vi "SpawnMediatorActor.vi"(6 "Unified Actor Alias":string, 9 "Core Leaf Actors":refnum<class "Actor.lvclass">[](array[class]), 10 "Actors":refnum<class "Actor.lvclass">[](array[class])) -> (0 "Error out":errorcluster, 2 "Root Unified Actor DVR":refnum<data-value>)   [LabVIEW 2020, in "jettl.lvlib"]
uses:
  jettl.lvlib
  Actor.ctl
  ActorLifetime.ctl
  Message/Message.lvclass
  MessageSet.ctl
  ActorRelation.ctl
  MessageMetadata.ctl
  Message.ctl
  Messages.ctl
  Actor/Actor.lvclass
  BaseActor/BaseActor.lvlib
  ActorType.ctl
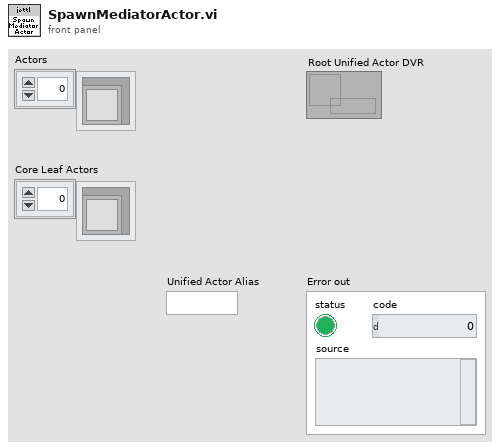
[diagram p1: front panel]
types:
  T1 = typedef "jettl.lvlib/Messages.ctl" = cluster{"Listen":T2, "Tell":T2, "TellSelf":T2, "TellActor":T2}
  T2 = typedef "jettl.lvlib/MessageSet.ctl" = set{refnum<class "Message.lvclass">}
  T3 = typedef "jettl.lvlib/Actor.ctl" = cluster{"Messages":T1, "Alias":string, "Transport":refnum<user-event>, "Address":refnum<event-registration>, "VIRef":refnum<vi>, "ActorType":T4}
  T4 = typedef "jettl.lvlib/ActorType.ctl" = enum16{"Mediator", "Component"}
  T5 = typedef "jettl.lvlib/ActorLifetime.ctl" = enum16{"Init", "Spawn", "Setup", "Teardown Before Running", "Running", "Stop Called", "Stopping With Children", "Stopping Without Children", "Teardown After Running", "Stopped"}
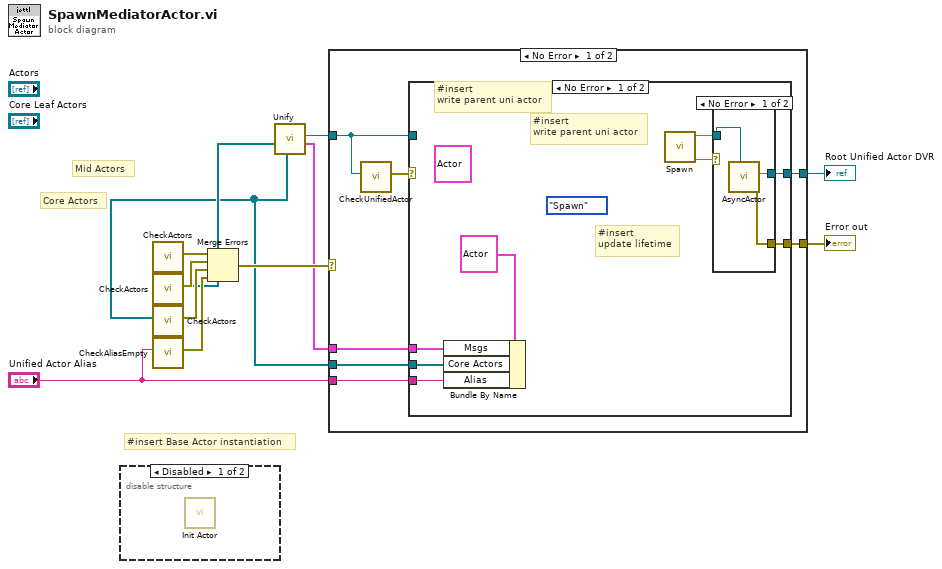
[diagram p0: block diagram]
diagram:
  # "Core Actors"
  # "Mid Actors"
  # "#insert Base Actor instantiation"
  n1 = disable-structure shown="Disabled" {
    frame Disabled {
      n2 = call "Init Actor.vi"() -> ()  [unwired: 11 in, 1 out]
    }
    frame Enabled {
    }
  }
  n3 = call "CheckActors.vi"() -> ("Error"=w7:errorcluster)  [unwired: 11 in]
  n4 = call "CheckActors.vi"() -> ("Error"=w11:errorcluster, "Actors"=w6:refnum<class "Actor.lvclass">[])  [unwired: 10 in]
  n5 = call "CheckActors.vi"() -> ("Error"=w8:errorcluster, "Actors"=w5:refnum<class "Actor.lvclass">[])  [unwired: 10 in]
  n6 = call "CheckAliasEmpty.vi"("Alias"="Unified Actor Alias") -> ("Error"=w10:errorcluster)  [unwired: 10 in]
  n7 = Merge Errors(w7, w11, w8, w10) -> (w12:errorcluster)
  n8 = call "Unify.vi"("Core Actors"=w5, "Mid Actors"=w6) -> ("Msgs"=w3:T1, "Unified Actor"=w2:refnum<class "Actor.lvclass">)  [unwired: 7 in, 1 out]
  n9 = case shown="No Error" w12 {
    selector: w12 -> [_ w37]
    tunnel: [w19 w37] -> w1
    tunnel: [w18 _] -> w4
    tunnel: "Unified Actor Alias" -> [w17 _]
    tunnel: w5 -> [w13 _]
    tunnel: w3 -> [w15 _]
    tunnel: w2 -> [w14 _]
    frame No Error {
      n10 = call "CheckUnifiedActor.vi"("Unified Actor"=w14) -> ("Error"=w16:errorcluster)  [unwired: 10 in]
      n11 = case shown="No Error" w16 {
        selector: w16 -> [_ w36]
        tunnel: [w31 w36] -> w19
        tunnel: [w30 _] -> w18
        tunnel: w17 -> [w29 _]
        tunnel: w15 -> [w27 _]
        tunnel: w14 -> [w22 _]
        tunnel: w13 -> [w23 _]
        frame No Error {
          w21 = ActorLifetime."Spawn" ("Lifetime")
          (unwired) T3 {"Messages"={"Listen"={}, "Tell"={}, "TellSelf"={}, "TellActor"={}}, "Alias"="", "Transport"=refnum, "Address"=refnum, "VIRef"=refnum, "ActorType"=enum."Mediator"} ("Parent Actor Attributes")
          # "#insert\nupdate lifetime"
          # "#insert\nwrite parent uni actor"
          # "#insert\nwrite parent uni actor"
          n12 = Bundle By Name(cluster=T3 {"Messages"={"Listen"={}, "Tell"={}, "TellSelf"={}, "TellActor"={}}, "Alias"="", "Transport"=refnum, "Address"=refnum, "VIRef"=refnum, "ActorType"=enum."Mediator"} ("Attributes"), "Msgs"=w27, "Core Actors"=w23, "Alias"=w29) -> (w26:T3)
          n13 = call-dynamic "Spawn.vi"() -> (0:w24, 3:w25, 11:w20)  [unwired: 7 in, 2 out]
          n14 = case shown="No Error" w24 {
            selector: w24 -> [_ w35]
            tunnel: [w34 w35] -> w31
            tunnel: [w33 _] -> w30
            tunnel: w25 -> [w32 _]
            frame No Error {
              n15 = call "AsyncActor.vi"("Actor in"=w32) -> ("Error out"=w34:errorcluster, 2:w33)  [unwired: 9 in]
            }
            frame Error {
            }
          }
        }
        frame Error {
        }
      }
    }
    frame Error {
    }
  }
  "Error out" <- w1
  "Root Unified Actor DVR" <- w4
